vi "bloc_turbocodage.vi"(11 "Array in":dbl[](array[numeric])) -> (1 "output bit stream":i8[](array[numeric]), 2 "sortie turbocodeur":string, 3 "sortie générateur":string)   [LabVIEW 2018]
uses:
  <vilib>/addons/Modulation/niDMT.lvlib
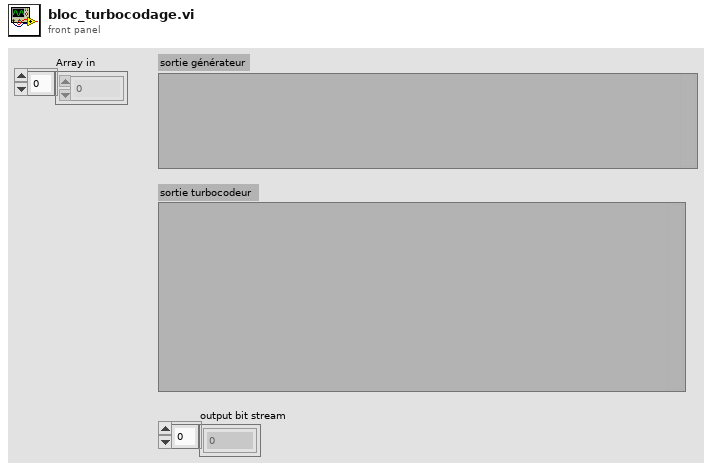
[diagram p1: front panel]
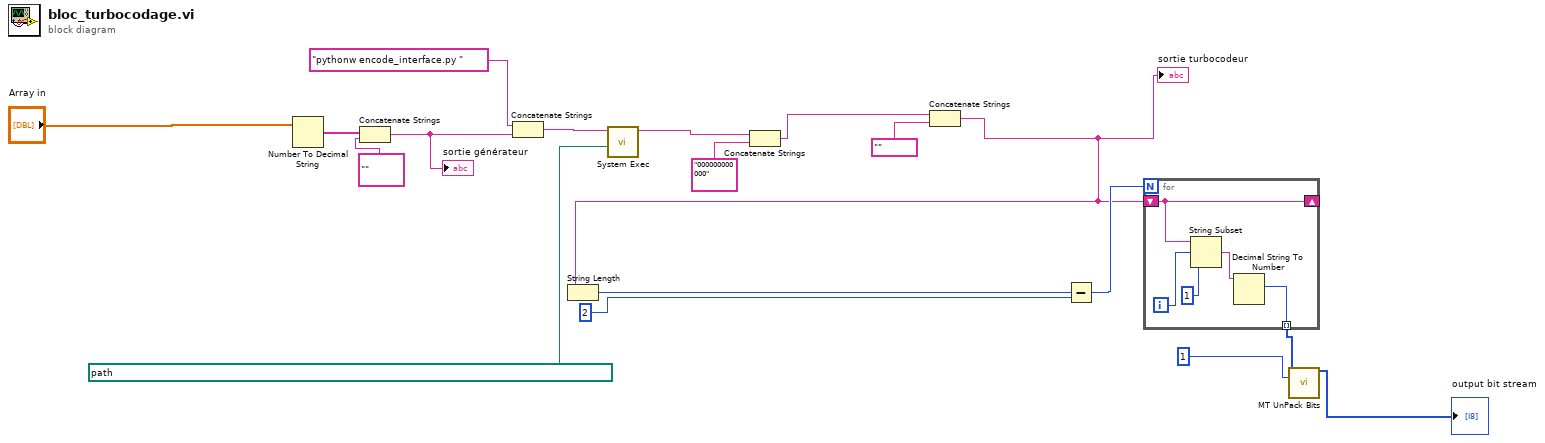
[diagram p0: block diagram]
diagram:
  n1 = Number To Decimal String(number="Array in") -> (decimal integer string=w17:string[])  [unwired: 1 in]
  n2 = Concatenate Strings(w17, "") -> (w15:string)
  "sortie générateur" <- w15
  n3 = Concatenate Strings("pythonw encode_interface.py ", w15) -> (w14:string)
  n4 = call <vilib>:"System Exec.vi"("working directory"=path "C:/Users/pc-labview/Desktop/Levi/Turbo-Codes/Implémentation perso Python/Turbocodes_OO", "command line"=w14) -> ("standard output"=w5:string)  [unwired: 4 in, 5 out]
  n5 = Concatenate Strings(w5, "000000000000") -> (w2:string)
  n6 = Concatenate Strings(w2, "") -> (w1:string)
  "sortie turbocodeur" <- w1
  n7 = String Length(string=w1) -> (length=w9:i32)
  n8 = Subtract(x=w9, y=2) -> (x-y=w10:i32)
  n9 = for {
    N: w10 -> [_]
    tunnel: [w20] -> w11 mode=indexing
    shift-right: [w19] -> _
    shift-left: w1 -> [w19]
    i -> [w23]
    n10 = String Subset(string=w19, offset (0)=w23, length (rest)=1) -> (substring=w21:string)
    n11 = Decimal String To Number(string=w21) -> (number=w20:i32)  [unwired: 2 in, 1 out]
  }
  n12 = call <vilib>:"MT UnPack Bits.vi"("input integers"=w11, "bits per integer"=1) -> ("output bit stream"=→"output bit stream":i8[])  [unwired: 12 in, 1 out]
